vi "Script BunUnbun IO Wire.vi"(4 "Wire Source":refnum<vi>[](array[refnum]), 6 "Indicator":bool, 8 "error in":errorcluster, 9 "VI":refnum<vi>, 10 "Terminal Attributes":T1) -> (0 "error out":errorcluster)   [LabVIEW 2020, in "_Rescript.lvlib" / "Msg.lvlib" / "Msg.lvclass"]
uses:
  Msg.lvclass
  _Rescript.lvlib
  Attributes.ctl
  Terminal Attributes.ctl
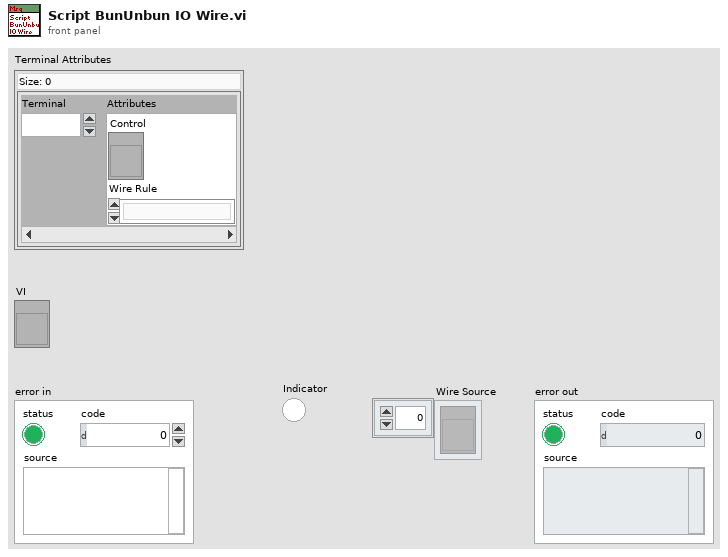
[diagram p1: front panel]
types:
  T1 = typedef "_Rescript.lvlib/Terminal Attributes.ctl" = map{i32, T2}
  T2 = typedef "_Rescript.lvlib/Attributes.ctl" = cluster{"Control":refnum<vi>, "Wire Rule":enum16{"Invalid Wire Rule", "Required", "Recommended", "Optional", "Dynamic Dispatch"}}
  T3 = enum16{"Invalid Wire Rule", "Required", "Recommended", "Optional", "Dynamic Dispatch"}
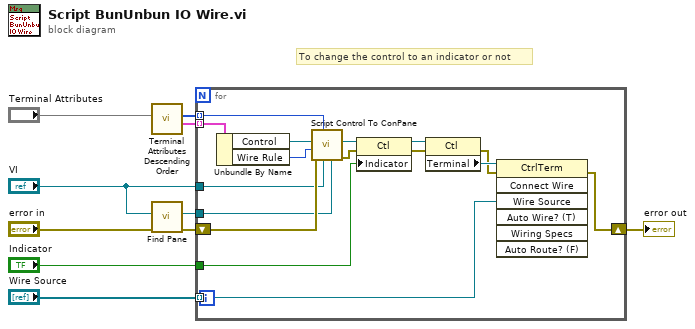
[diagram p0: block diagram]
diagram:
  # "To change the control to an indicator or not"
  n1 = call "Terminal Attributes Descending Order.vi"("Terminal Attributes"="Terminal Attributes") -> ("Attributes Descending Order"=w8:T2[], "Terminal Descending Order"=w7:i32[])  [unwired: 9 in]
  n2 = call "Find Pane.vi"("error in"="error in", "VI"="VI") -> ("error out"=w10:errorcluster, "Pane Ref"=w9:refnum<vi>)  [unwired: 8 in]
  n3 = for {
    tunnel: w7 -> [w15] mode=indexing
    tunnel: w9 -> [w22]
    tunnel: "VI" -> [w16]
    shift-right: [w24] -> w5
    shift-left: w10 -> [w23]
    tunnel: w8 -> [w13] mode=indexing
    tunnel: "Indicator" -> [w12]
    tunnel: "Wire Source" -> [w11] mode=indexing
    n4 = Unbundle By Name(w13) -> ("Control"=w21:refnum<vi>, "Wire Rule"=w20:T3)
    n5 = call "Script Control To ConPane.vi"("Pane"=w22, "VI"=w16, "Terminal"=w15, "error in"=w23, "Wire Rule"=w20, "Control To Duplicate"=w21) -> ("error out"=w18:errorcluster, "Duplicated Control"=w19:refnum<vi>)  [unwired: 4 in]
    n6 = property class="Ctl"(reference=w19, error in=w18, "Indicator"=w12) -> (reference out=w17:refnum<vi>, error out=w14:errorcluster)
    n7 = property class="Ctl"(reference=w17, error in=w14) -> (error out=w25:errorcluster, "Terminal"=w26:refnum<vi>)  [unwired: 1 out]
    n8 = invoke class="CtrlTerm" method="Connect Wire"(reference=w26, error in=w25, "Wire Source"=w11) -> (error out=w24:errorcluster)  [unwired: 4 in, 6 out]
  }
  "error out" <- w5
